vi "FGV - KeyFocus.vi"(7 "Action":T1, 8 "error in (no error)":errorcluster, 11 "VI ref":refnum<vi>) -> (0 "error out":errorcluster, 3 "input VI ref = Focus?":bool)   [LabVIEW 2021, in "RocketPlot.lvlib"]
uses:
  RocketPlot.lvlib
  TypeDefs/FGV - KeyFocus action.ctl
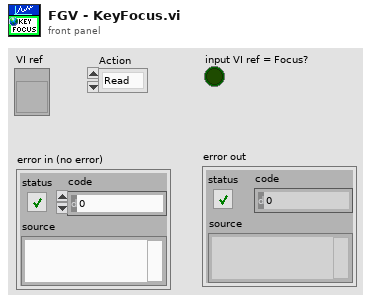
[diagram p1: front panel]
types:
  T1 = typedef "RocketPlot.lvlib/FGV - KeyFocus action.ctl" = enum16{"Read", "Write", "Clear"}
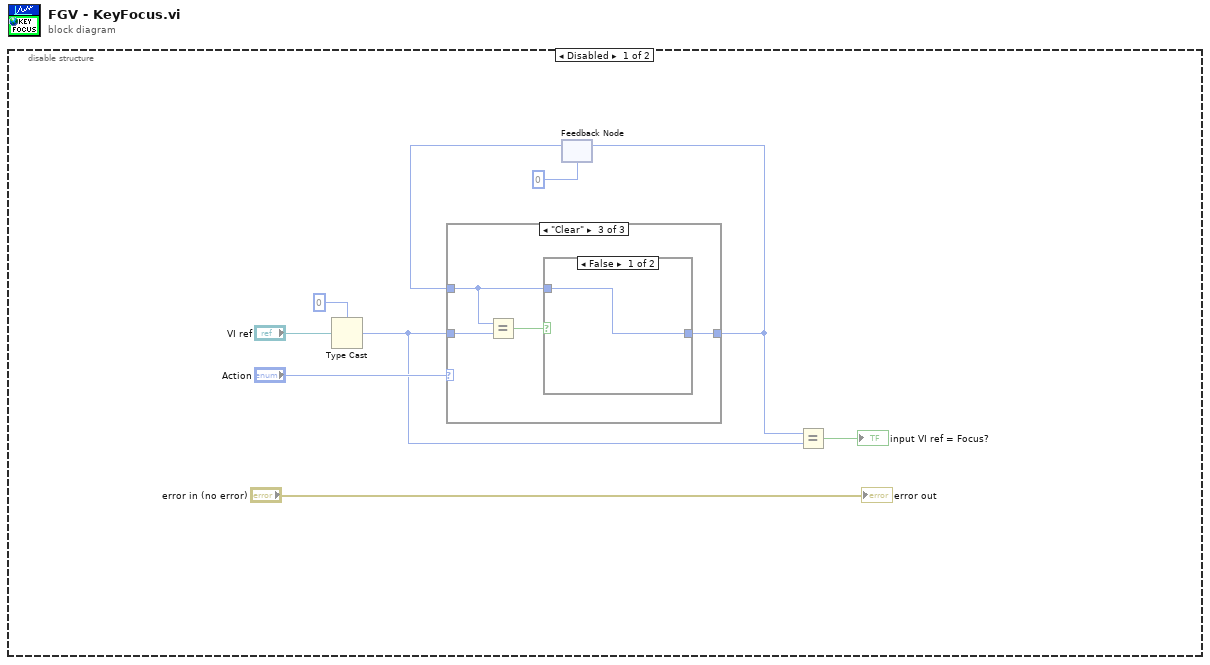
[diagram p0: block diagram]
diagram:
  n1 = disable-structure shown="Disabled" {
    frame Disabled {
      n2 = Type Cast(type=u32 0 ("unsigned 32bit integer"), x="VI ref") -> (*(type *) &x=w3:u32)
      n3 = feedback #1(u32 0 ("unsigned 32bit integer")) -> (w9:u32)
      n4 = case shown="\"Clear\"" "Action" {
        tunnel: [w10 w11 w13] -> w4
        tunnel: w3 -> [_ w11 w15]
        tunnel: w9 -> [w10 _ w12]
        frame "Read" {
        }
        frame "Write" {
        }
        frame "Clear" {
          n5 = Equal?(x=w12, y=w15) -> (x = y?=w14:bool)
          n6 = case shown="False" w14 {
            tunnel: [w16 _] -> w13
            tunnel: w12 -> [w16 _]
            frame False {
            }
            frame True {
            }
          }
        }
      }
      n7 = feedback-in #1(w4) -> ()
      n8 = Equal?(x=w4, y=w3) -> (x = y?=→"input VI ref = Focus?":bool)
      "error out" <- "error in (no error)"
    }
    frame Enabled {
    }
  }
